vi "Timed Actor Message.vi"(9 "Interval (ms)":u32, 10 "Message":refnum<class "Message.lvclass">, 11 "Message Queue":refnum<queue>) -> ()   [LabVIEW 2026]
uses:
  Parent Classes/Message/Message.lvclass
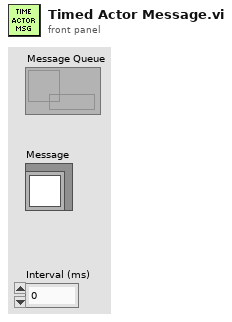
[diagram p1: front panel]
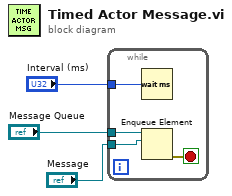
[diagram p0: block diagram]
diagram:
  n1 = while {
    tunnel: "Interval (ms)" -> [w6]
    tunnel: "Message" -> [w5]
    tunnel: "Message Queue" -> [w4]
    stop <- w7 stop-if-true
    n2 = Wait (ms)(milliseconds to wait=w6) -> ()  [unwired: 1 out]
    n3 = Enqueue Element(queue=w4, element=w5) -> (error out=w7:errorcluster)  [unwired: 2 in, 2 out]
  }
